vi "Folder Hierarchy Verifier.vi"() -> ()   [LabVIEW 2023]
doc: "Presents an interface to view the expected folder hierarchy on disk and and compare it to the actual folder hierarchy."
uses:
  CTLs/Folder Verifier State Data.ctl
  <userlib>/_MGI/Application Control/MGI Gray if/MGI Gray if False.vi
  SubVIs/FaKI State Machine/FaKI State Machine.lvlib
panel:
  in  "Project Hierarchy":string(tree)
  in  "Analyze Project":bool
  in  "Exit":bool
  in  "Project File":path
  # "A non-container project item will be red if expected path does not match actual path. A container project item will be red if none of the containing expected paths match actual paths, and purple if some match and some don't match"
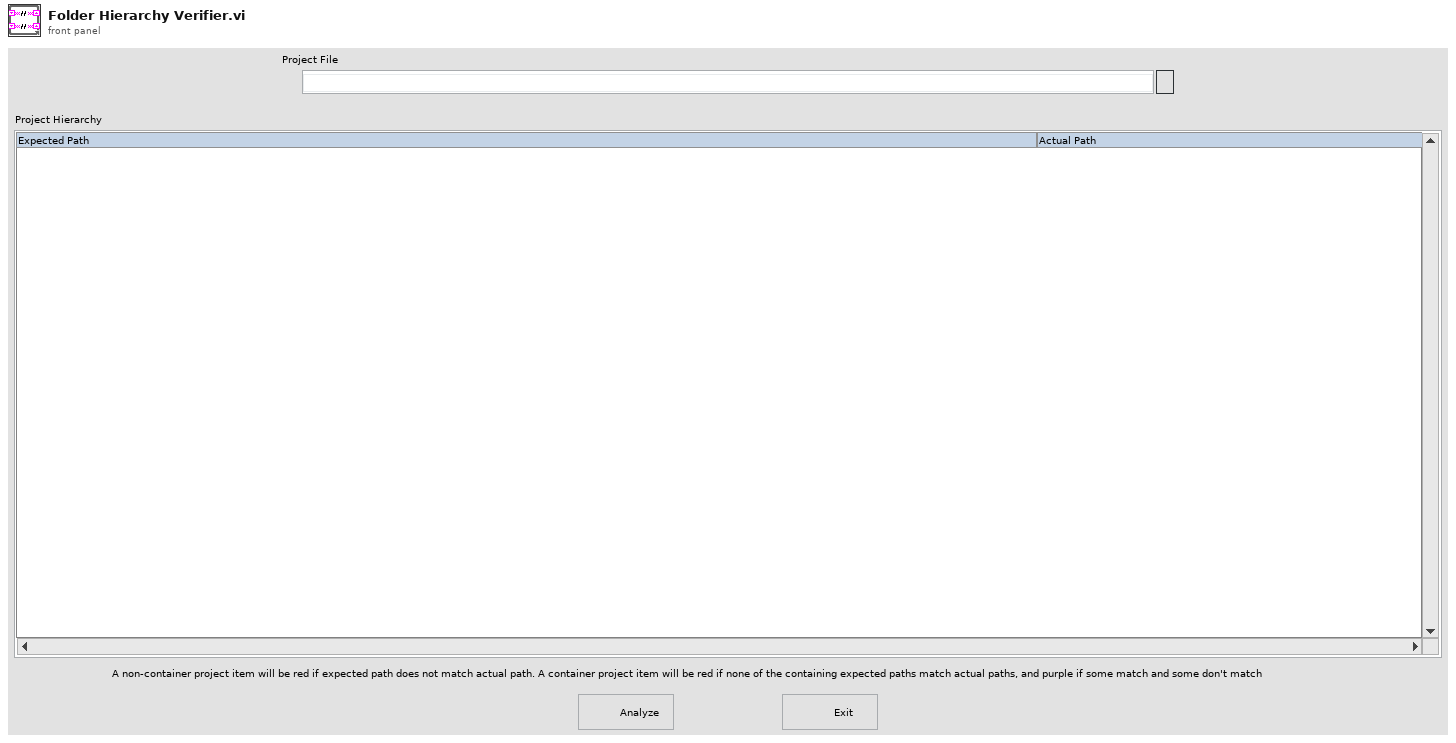
[diagram p1: front panel]
types:
  T1 = typedef "Folder Verifier State Data.ctl" = cluster{"Core":cluster{"Current VI Reference":refnum<vi>, "Close Panel on Exit?":bool}, "Tree Refnum":refnum<vi>, "Project":path, "Expected Paths":path[], "Actual Paths":path[]}
  T2 = enum32{"Invalid", "Standard", "Closed", "Hidden", "Minimized", "Maximized"}
  T3 = enum32{"invalid app kind", "Development System", "Run Time System", "Student Edition", "Embedded LabVIEW", "Evaluation", "Custom"}
  T4 = enum8{"Enabled", "Disabled", "Disabled and Grayed Out"}
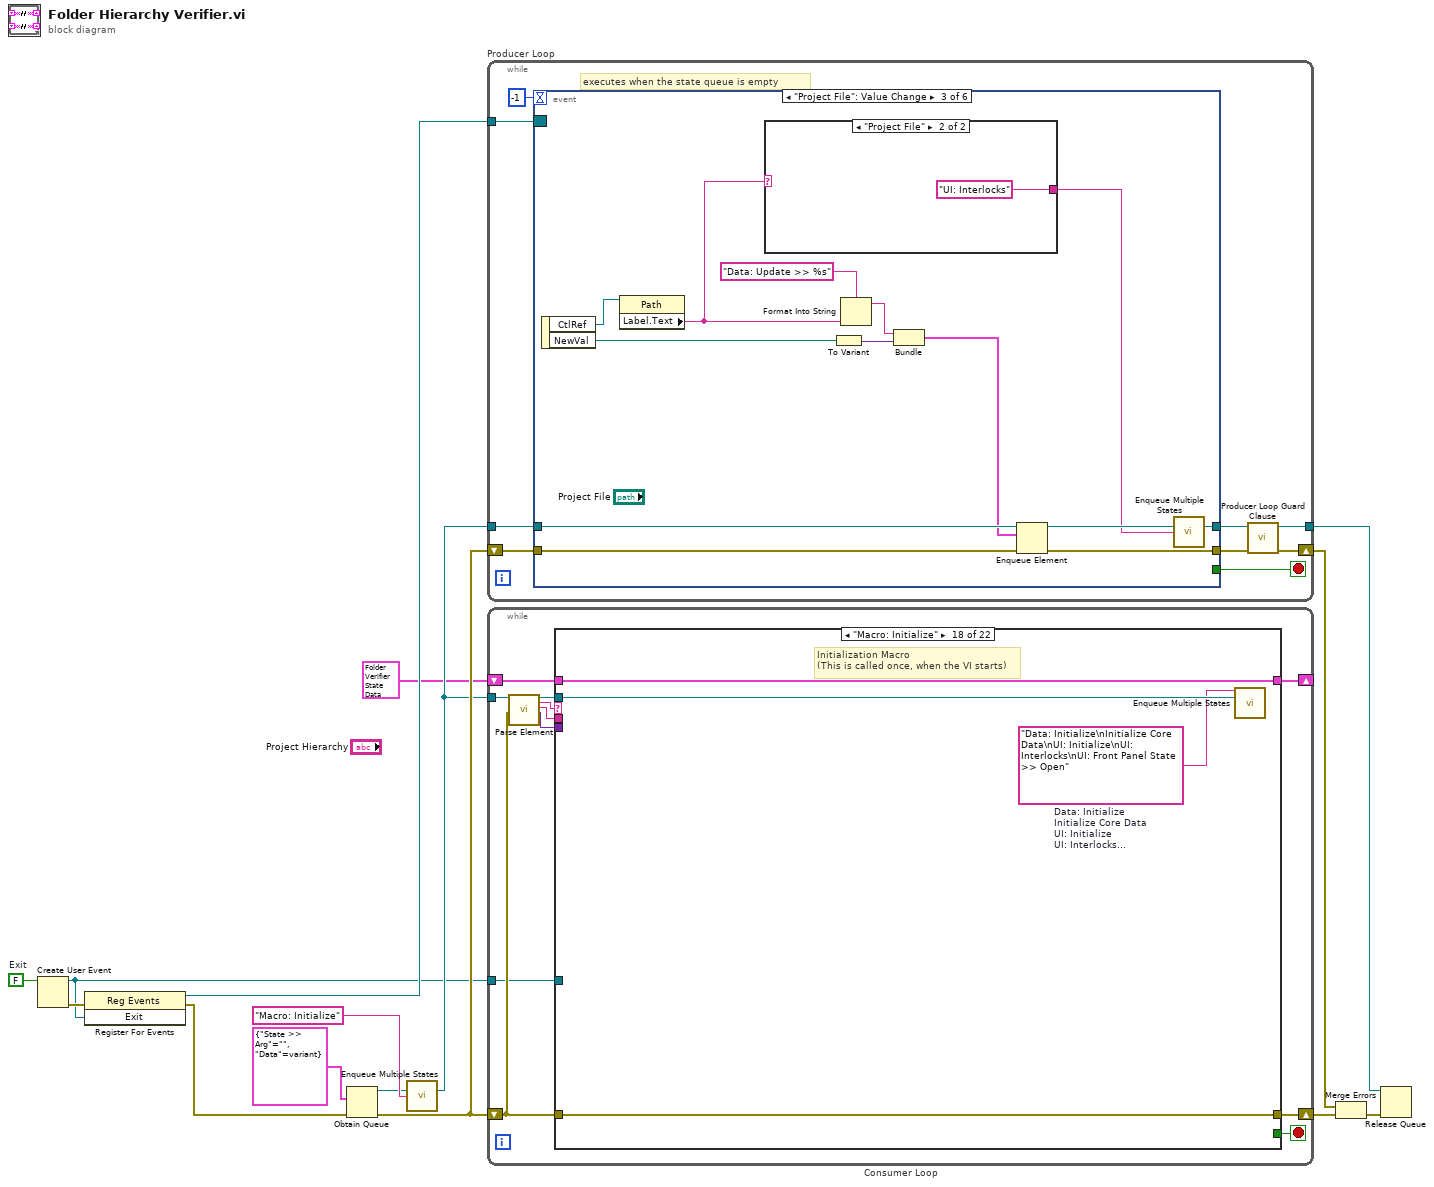
[diagram p0: block diagram]
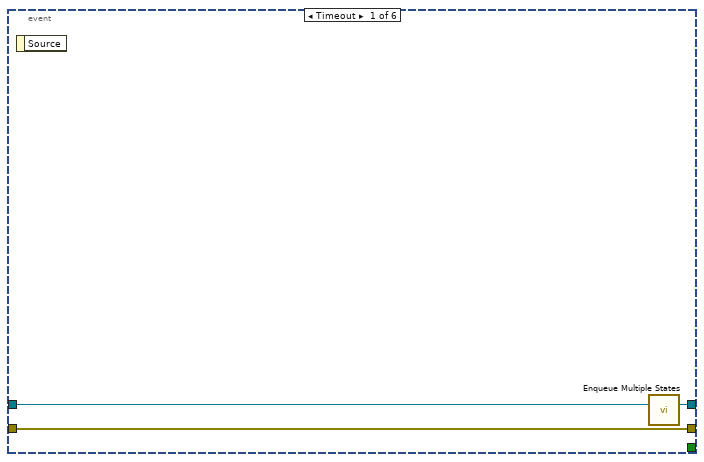
[diagram p2: hidden frame]
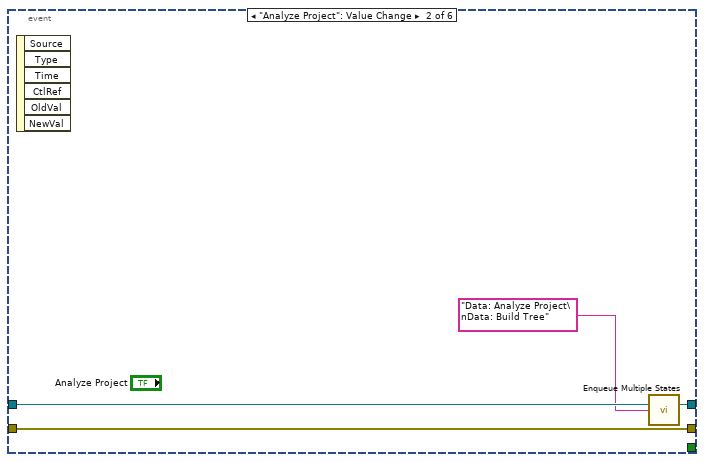
[diagram p3: hidden frame]
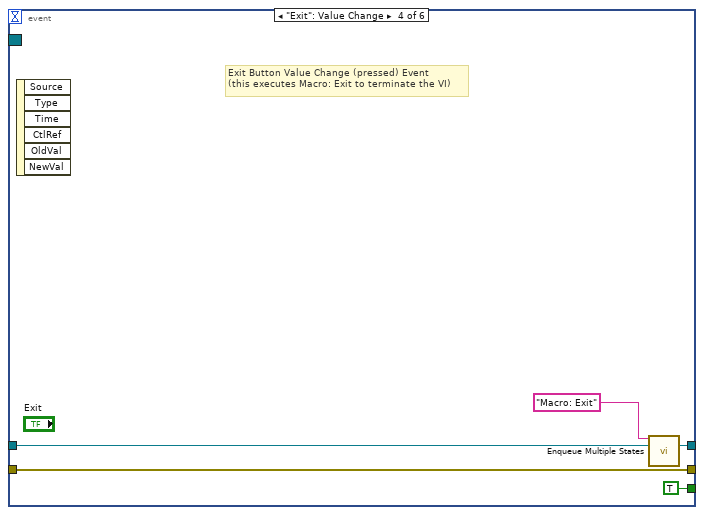
[diagram p5: hidden frame]
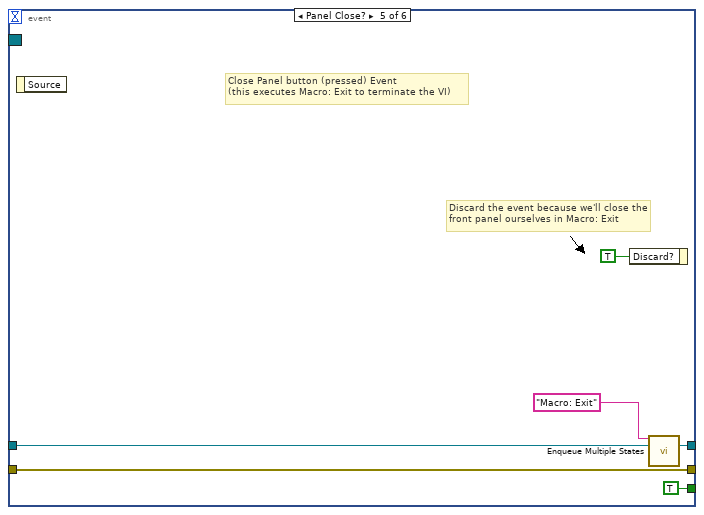
[diagram p6: hidden frame]
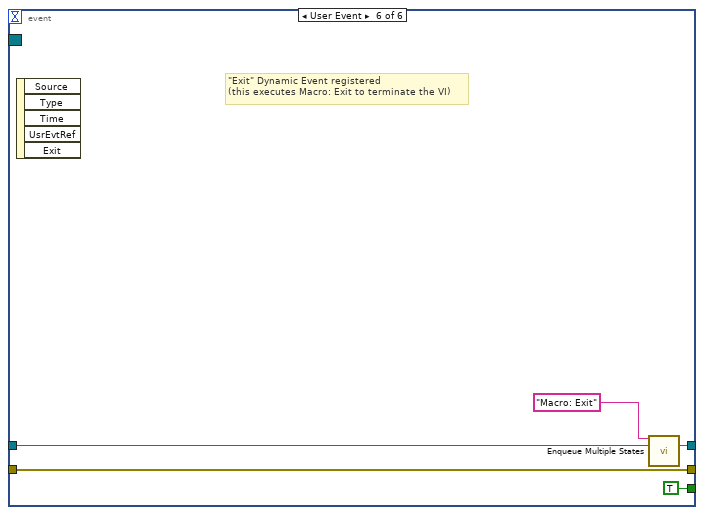
[diagram p7: hidden frame]
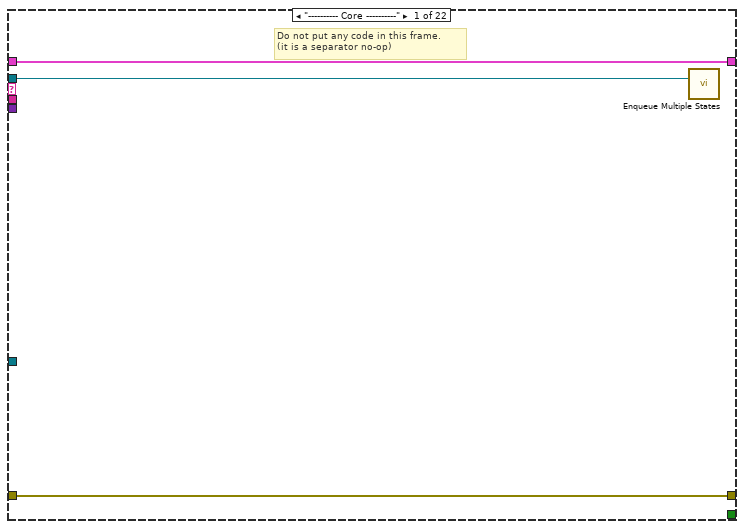
[diagram p8: hidden frame]
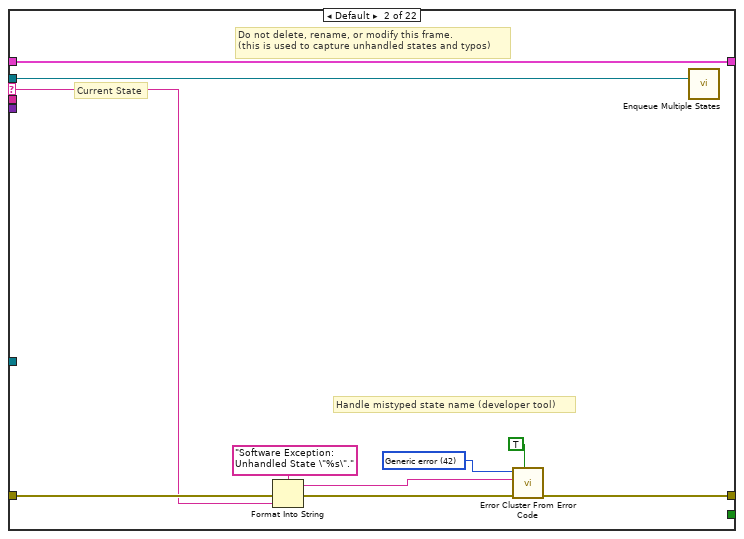
[diagram p9: hidden frame]
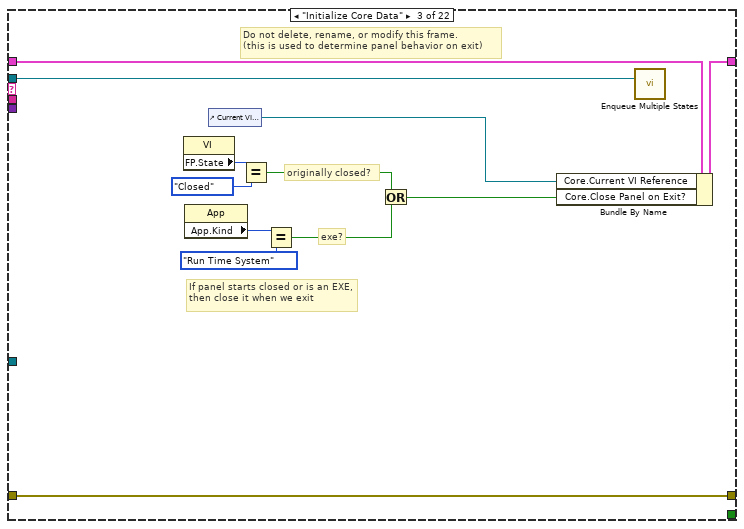
[diagram p10: hidden frame]
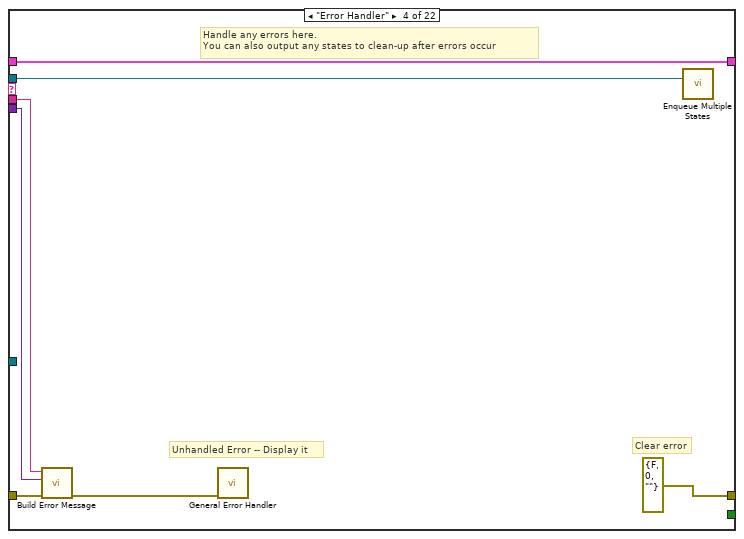
[diagram p11: hidden frame]
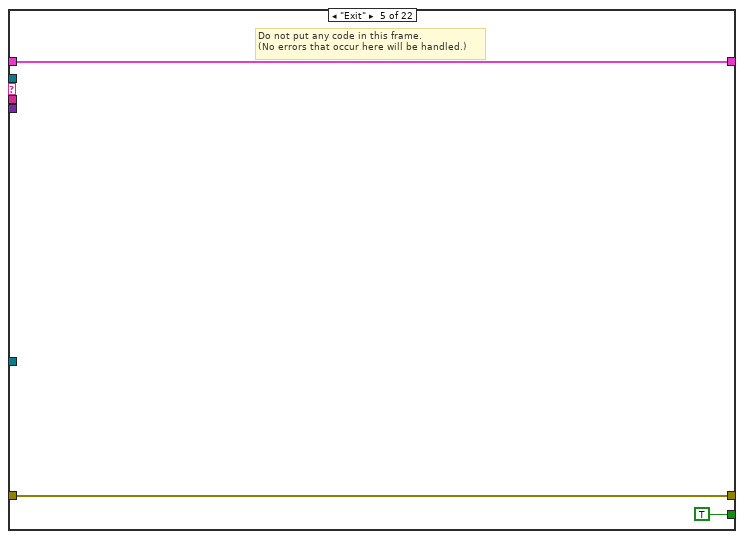
[diagram p12: hidden frame]
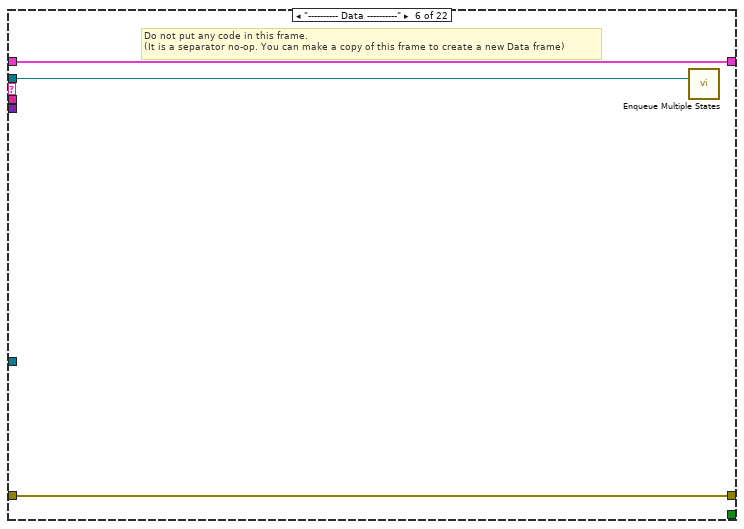
[diagram p13: hidden frame]
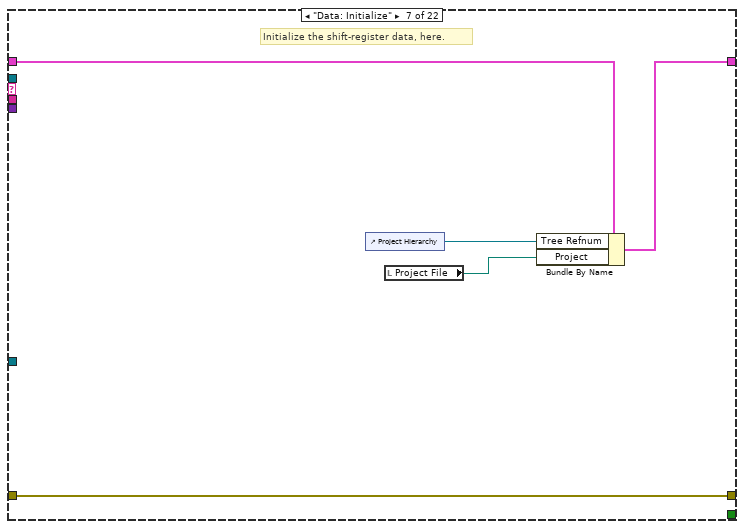
[diagram p14: hidden frame]
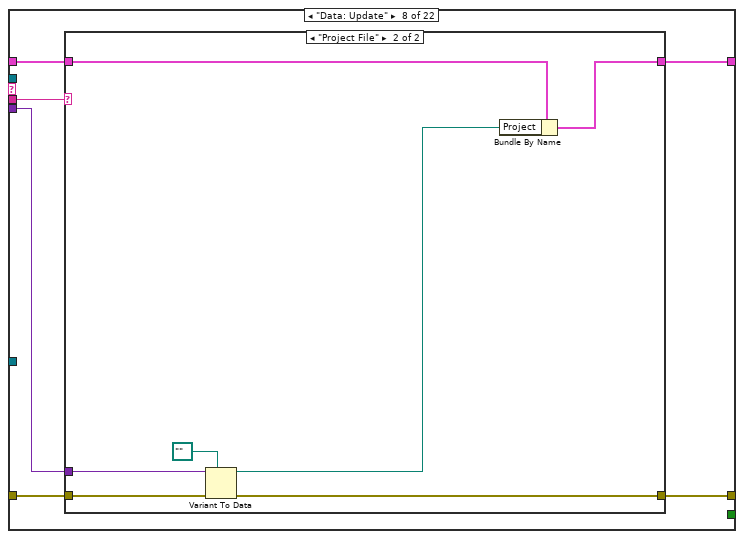
[diagram p15: hidden frame]
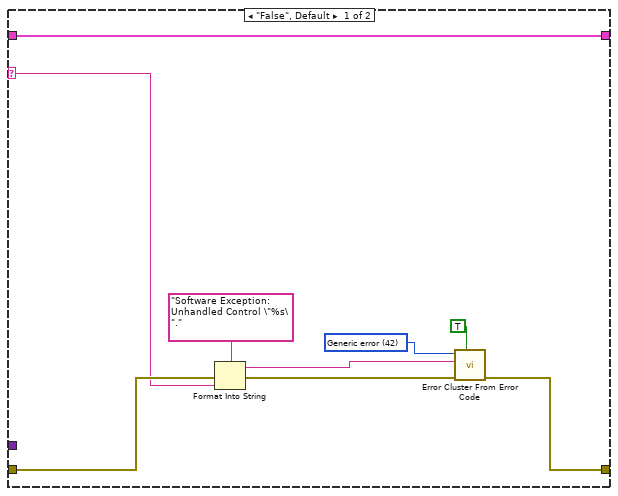
[diagram p16: hidden frame]
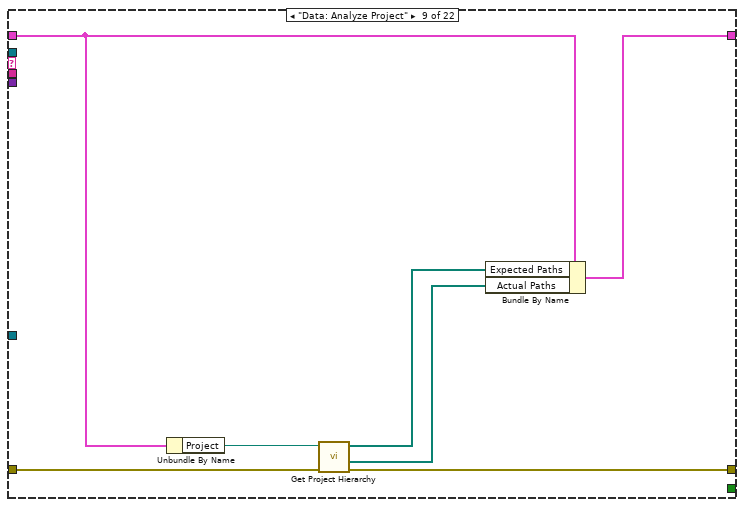
[diagram p17: hidden frame]
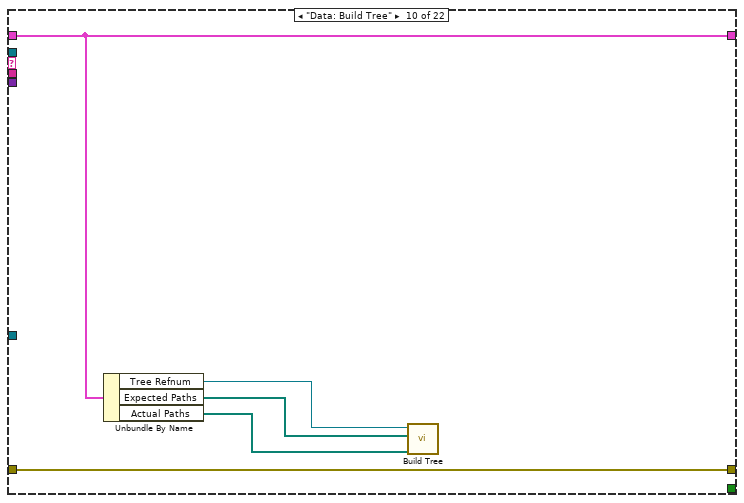
[diagram p18: hidden frame]
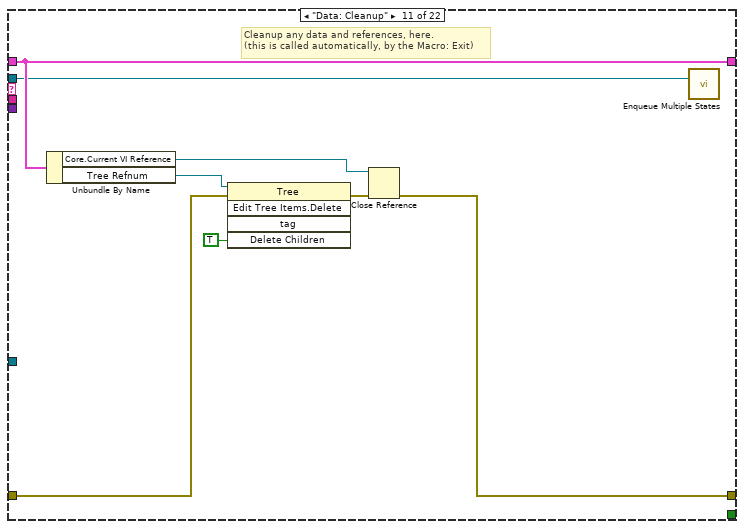
[diagram p19: hidden frame]
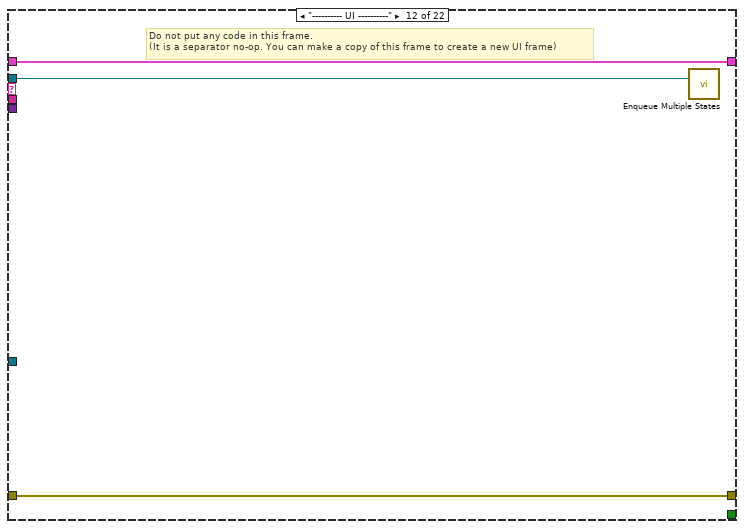
[diagram p20: hidden frame]
diagram:
  w5 = FALSE  # Exit
  n1 = Create User Event(user event datatype=w5) -> (user event=w2:refnum<user-event>, error out=w6:errorcluster)  [unwired: 1 in]
  n2 = register-events(error in=w6, w2) -> (reference out=w3:refnum<event-registration>, error out=w4:errorcluster)  [unwired: 1 in]
  n3 = Obtain Queue(element data type=cluster{"State >> Arg":string, "Data":variant} {"State >> Arg"="", "Data"=variant}, error in (no error)=w4) -> (queue out=w12:refnum<queue>, error out=w15:errorcluster)  [unwired: 3 in, 1 out]
  n4 = call "Enqueue Multiple States.vi"("queue in"=w12, "State(s) at Back"="Macro: Initialize") -> ("queue out"=w11:refnum<queue>)  [unwired: 13 in]
  n5 = while "Producer Loop" {
    shift-right: [w19] -> w9
    shift-left: w15 -> [w24]
    tunnel: w3 -> [w16]
    tunnel: w11 -> [w22]
    tunnel: [w17] -> w7
    stop <- w21 stop-if-true
    # "executes when the state queue is empty"
    n6 = event shown="[2] \"Project File\": Value Change" {
      selector: w16 -> [_ _ _ _ _ _]
      dyn-events: _ -> [_ _ _ _ _ _]
      timeout: -1 ("Timeout") -> [_ _ _ _ _ _]
      tunnel: [w25 w29 w42 w50 w56 w61] -> w20
      tunnel: w24 -> [w25 w29 w43 w50 w56 w61]
      tunnel: w22 -> [w26 w30 w41 w49 w53 w59]
      tunnel: [w27 w31 w44 w47 w52 w58] -> w18
      tunnel: [_ _ _ TRUE TRUE TRUE] -> w21
      event Timeout {
        n7 = event-data() -> ()  [unwired: 1 in, 1 out]
        n8 = call "Enqueue Multiple States.vi"("queue in"=w26) -> ("queue out"=w27:refnum<queue>)  [unwired: 14 in]
      }
      event "Analyze Project": Value Change {
        n9 = event-data() -> ()  [unwired: 1 in, 6 out]
        n10 = call "Enqueue Multiple States.vi"("queue in"=w30, "State(s) at Back"="Data: Analyze Project\nData: Build Tree") -> ("queue out"=w31:refnum<queue>)  [unwired: 13 in]
      }
      event "Project File": Value Change {
        n11 = event-data() -> ("CtlRef"=w39:refnum<vi>, "NewVal"=w38:path)  [unwired: 1 in]
        n12 = property class="Path"(reference=w39) -> ("Label.Text"=w34:string)  [unwired: 1 in, 2 out]
        n13 = case shown="\"Project File\"" w34 {
          tunnel: [_ "UI: Interlocks"] -> w32
          frame "False", Default {
          }
          frame "Project File" {
          }
        }
        n14 = To Variant(anything=w38) -> (Variant=w37:variant)
        n15 = Format Into String(format string="Data: Update >> %s", w34) -> (resulting string=w36:string)  [unwired: 2 in, 1 out]
        n16 = Bundle(w36, "Variant"=w37) -> (w33:cluster{string, "Variant":variant})  [unwired: 1 in]
        n17 = Enqueue Element(queue=w41, element=w33, error in (no error)=w43) -> (queue out=w40:refnum<queue>, error out=w42:errorcluster)  [unwired: 1 in, 1 out]
        n18 = call "Enqueue Multiple States.vi"("queue in"=w40, "State(s) at Back"=w32) -> ("queue out"=w44:refnum<queue>)  [unwired: 13 in]
      }
      event "Exit": Value Change {
        # "Exit Button Value Change (pressed) Event\n(this executes Macro: Exit to terminate the VI)"
        n19 = event-data() -> ()  [unwired: 1 in, 6 out]
        n20 = call "Enqueue Multiple States.vi"("State(s) at Front"="Macro: Exit", "queue in"=w49) -> ("queue out"=w47:refnum<queue>)  [unwired: 13 in]
      }
      event Panel Close? {
        # "Discard the event because we'll close the front panel ourselves in Macro: Exit"
        # "Close Panel button (pressed) Event\n(this executes Macro: Exit to terminate the VI)"
        n21 = event-data() -> ()  [unwired: 1 in, 1 out]
        n22 = event-data("Discard?"=TRUE) -> ()  [unwired: 1 in, 1 out]
        n23 = call "Enqueue Multiple States.vi"("State(s) at Front"="Macro: Exit", "queue in"=w53) -> ("queue out"=w52:refnum<queue>)  [unwired: 13 in]
      }
      event User Event {
        # "\"Exit\" Dynamic Event registered\n(this executes Macro: Exit to terminate the VI)"
        n24 = event-data() -> ()  [unwired: 1 in, 5 out]
        n25 = call "Enqueue Multiple States.vi"("State(s) at Front"="Macro: Exit", "queue in"=w59) -> ("queue out"=w58:refnum<queue>)  [unwired: 13 in]
      }
    }
    n26 = call "Producer Loop Guard Clause.vi"("error in (no error)"=w20, "queue in"=w18) -> ("error out"=w19:errorcluster, "queue out"=w17:refnum<queue>)  [unwired: 8 in]
  }
  n27 = while "Consumer Loop" {
    shift-right: [w69] -> _
    shift-left: T1 {"Core"={"Current VI Reference"=refnum, "Close Panel on Exit?"=FALSE}, "Tree Refnum"=refnum, "Project"=path "", "Expected Paths"=[], "Actual Paths"=[]} ("Folder Verifier State Data") -> [w68]
    shift-right: [w72] -> w10
    shift-left: w15 -> [w71]
    tunnel: w11 -> [w67]
    tunnel: w2 -> [w62]
    stop <- w70 stop-if-true
    n28 = call "Parse Element.vi"("queue in"=w67, "error in (no error)"=w71) -> ("queue out"=w66:refnum<queue>, "State"=w65:string, "Arg"=w64:string, "Data"=w63:variant)  [unwired: 14 in]
    n29 = case shown="\"Macro: Initialize\"" w65 {
      selector: w65 -> [_ w77 _ _ _ _ _ _ _ _ _ _ _ _ _ _ _ _ _ _ _ _]
      tunnel: w66 -> [w73 w76 w86 w102 _ w108 _ _ _ _ w154 w158 w161 _ w170 w179 w250 w254 w260 w266 w269 w272]
      tunnel: w64 -> [_ _ _ w98 _ _ _ w119 _ _ _ _ _ _ w171 w180 _ _ _ _ _ _]
      tunnel: w68 -> [w74 w79 w92 w103 w106 w109 w114 w120 w139 w149 w155 w159 w162 w168 w172 w182 w251 w255 w264 w267 w270 w273]
      tunnel: [w75 w84 w97 errorcluster {"status"=FALSE, "code"=0, "source"=""} ("error out") w107 w110 w115 w117 w143 w148 w157 w160 w163 w169 w173 w183 w252 w256 w265 w268 w271 w274] -> w72
      tunnel: w71 -> [w75 w83 w97 w101 w107 w110 w115 w121 w144 w148 w151 w160 w163 w169 w174 w184 w252 w256 w265 w268 w271 w274]
      tunnel: [_ _ _ _ TRUE _ _ _ _ _ _ _ _ _ _ _ _ _ _ _ _ _] -> w70
      tunnel: [w74 w79 w96 w103 w106 w109 w113 w116 w142 w149 w155 w159 w162 w168 w172 w182 w251 w255 w264 w267 w270 w273] -> w69
      tunnel: w63 -> [_ _ _ w99 _ _ _ w118 _ _ _ _ _ _ _ _ _ _ _ _ _ _]
      tunnel: w62 -> [_ _ _ _ _ _ _ _ _ _ _ _ _ _ _ _ _ _ _ _ _ _]
      frame "---------- Core ----------" {
        # "Do not put any code in this frame.\n(it is a separator no-op)"
        n30 = call "Enqueue Multiple States.vi"("queue in"=w73) -> ()  [unwired: 14 in, 1 out]
      }
      frame Default {
        w81 = 42 items=["No error", "Argument error", "Memory is full", "Out of zone", "End of file", "File already open", "Generic file I/O error", "File not found", "File permission error", "Disk is full", "Duplicate path", "Too many files open", "System feature not enabled", "Resource file not found", "Cannot add resource", "Resource not found", "Image not found", "Image memory error", "Pen does not exist", "Config type invalid", "Config token not found", "Config parse error", "Config memory error", "Bad external code format", "Bad external code offset", "External code not present", "Null window", "Destroy window error", "Null menu", "Print aborted", "Bad print record", "Print driver error", "Windows error during printing", "Memory error during printing", "Print dialog error", "Generic print error", "Invalid device refnum", "Device not found", "Device parameter error", "Device unit error", "Cannot open device", "Device call aborted", "Generic error", "Cancelled by user", "Object ID too low", "Object ID too high", "Object not in heap", "Unknown heap", "Unknown object (invalid DefProc)", "Unknown object (DefProc not in table)", "Message out of range", "Invalid (null) method", "Unknown message", "Manager call not supported", "Bad address", "Network operation in progress", "Network operation timed out", "Connection is busy", "Network attribute not supported", "Network error", "Address in use", "System out of memory", "Connection aborted", "Connection refused", "Not connected", "Already connected", "Connection closed", "Initialization error (interapplication manager)", "Bad occurrence", "Wait on unbound occurrence handler", "Occurrence queue overflow", "Datalog type conflict", "Unused", "Unrecognized type (interapplication manager)", "Memory corrupt", "Failed to make temporary DLL", "Old CIN version", "Drag socket not found", "Failed to load drop-object", "Failed to register OLE object", "Failed to release OLE object", "Format specifier type mismatch", "Unknown format specifier", "Too few format specifiers", "Too many format specifiers", "Scan failed", "Newer CIN version", "Error converting to variant", "Runtime menu error", "Password tampered", "Variant attribute not found", "Incompatible variant data type", "Event data is not available", "Event Store is not present", "Occurrence is not found", "Event Queue is not created", "Event info is not available", "Refnum passed is NULL", "Error retrieving Class GUID", "Error retrieving CoClass GUID", "Error retrieving TypeLib GUID.", "Bad built application magic bytes.", "Specific driver is different from the specific driver associated with the Logical Name.", "There is no session opened to the class driver.", "Max Error", "MAX - Error with config objects", "MAX - Error loading configuration", "MAX - Group not supported"]
        # "Current State"
        # "Do not delete, rename, or modify this frame.\n(this is used to capture unhandled states and typos)"
        # "Handle mistyped state name (developer tool)"
        n31 = Format Into String(format string="Software Exception: Unhandled State \"%s\"." ("message"), error in=w83, w77) -> (resulting string=w80:string, error out=w85:errorcluster)  [unwired: 1 in]
        n32 = call <vilib>:"Error Cluster From Error Code.vi"("show call chain? (False)"=TRUE, "error in (no error)"=w85, "error message (\"\")"=w80, "error code (0)"=w81) -> ("error out"=w84:errorcluster)  [unwired: 5 in]
        n33 = call "Enqueue Multiple States.vi"("queue in"=w76) -> ()  [unwired: 14 in, 1 out]
      }
      frame "Initialize Core Data" {
        # "Do not delete, rename, or modify this frame.\n(this is used to determine panel behavior on exit)"
        # "originally closed?"
        # "exe?"
        # "If panel starts closed or is an EXE, then close it when we exit"
        n34 = property class="VI"() -> ("FP.State"=w89:T2)  [unwired: 2 in, 2 out]
        n35 = property class="App"() -> ("App.Kind"=w95:T3)  [unwired: 2 in, 2 out]
        n36 = control-ref of="Current VI Reference"() -> (w90:refnum<vi>)
        n37 = Equal?(x=w89, y=T2."Closed" ("Front Panel Window:State")) -> (x = y?=w87:bool)
        n38 = Equal?(x=w95, y=T3."Run Time System" ("Application:Kind")) -> (x = y?=w93:bool)
        n39 = Or(x=w87, y=w93) -> (x .or. y?=w91:bool)
        n40 = Bundle By Name(cluster=w92, "Core.Current VI Reference"=w90, "Core.Close Panel on Exit?"=w91) -> (w96:T1)
        n41 = call "Enqueue Multiple States.vi"("queue in"=w86) -> ()  [unwired: 14 in, 1 out]
      }
      frame "Error Handler" {
        # "Unhandled Error -- Display it"
        # "Handle any errors here.\nYou can also output any states to clean-up after errors occur"
        # "Clear error"
        n42 = call "Build Error Message.vi"("error in (no error)"=w101, "Data"=w99, "Arg"=w98) -> ("error out"=w100:errorcluster)  [unwired: 8 in]
        n43 = call <vilib>:"General Error Handler.vi"("error in (no error)"=w100) -> ()  [unwired: 10 in, 5 out]
        n44 = call "Enqueue Multiple States.vi"("queue in"=w102) -> ()  [unwired: 14 in, 1 out]
      }
      frame "Exit" {
        # "Do not put any code in this frame.\n(No errors that occur here will be handled.)"
      }
      frame "---------- Data ----------" {
        # "Do not put any code in this frame.\n(It is a separator no-op. You can make a copy of this frame to create a new Data frame)"
        n45 = call "Enqueue Multiple States.vi"("queue in"=w108) -> ()  [unwired: 14 in, 1 out]
      }
      frame "Data: Initialize" {
        # "Initialize the shift-register data, here."
        n46 = control-ref of="Project Hierarchy"() -> (w112:refnum<vi>)
        n47 = local read "Project File"() -> (w111:path)
        n48 = Bundle By Name(cluster=w114, "Tree Refnum"=w112, "Project"=w111) -> (w113:T1)
      }
      frame "Data: Update" {
        n49 = case shown="\"Project File\"" w119 {
          selector: w119 -> [w122 _]
          tunnel: w121 -> [w124 w136]
          tunnel: w120 -> [w130 w133]
          tunnel: w118 -> [_ w137]
          tunnel: [w123 w134] -> w117
          tunnel: [w130 w132] -> w116
          frame "False", Default {
            w128 = 42 items=["No error", "Argument error", "Memory is full", "Out of zone", "End of file", "File already open", "Generic file I/O error", "File not found", "File permission error", "Disk is full", "Duplicate path", "Too many files open", "System feature not enabled", "Resource file not found", "Cannot add resource", "Resource not found", "Image not found", "Image memory error", "Pen does not exist", "Config type invalid", "Config token not found", "Config parse error", "Config memory error", "Bad external code format", "Bad external code offset", "External code not present", "Null window", "Destroy window error", "Null menu", "Print aborted", "Bad print record", "Print driver error", "Windows error during printing", "Memory error during printing", "Print dialog error", "Generic print error", "Invalid device refnum", "Device not found", "Device parameter error", "Device unit error", "Cannot open device", "Device call aborted", "Generic error", "Cancelled by user", "Object ID too low", "Object ID too high", "Object not in heap", "Unknown heap", "Unknown object (invalid DefProc)", "Unknown object (DefProc not in table)", "Message out of range", "Invalid (null) method", "Unknown message", "Manager call not supported", "Bad address", "Network operation in progress", "Network operation timed out", "Connection is busy", "Network attribute not supported", "Network error", "Address in use", "System out of memory", "Connection aborted", "Connection refused", "Not connected", "Already connected", "Connection closed", "Initialization error (interapplication manager)", "Bad occurrence", "Wait on unbound occurrence handler", "Occurrence queue overflow", "Datalog type conflict", "Unused", "Unrecognized type (interapplication manager)", "Memory corrupt", "Failed to make temporary DLL", "Old CIN version", "Drag socket not found", "Failed to load drop-object", "Failed to register OLE object", "Failed to release OLE object", "Format specifier type mismatch", "Unknown format specifier", "Too few format specifiers", "Too many format specifiers", "Scan failed", "Newer CIN version", "Error converting to variant", "Runtime menu error", "Password tampered", "Variant attribute not found", "Incompatible variant data type", "Event data is not available", "Event Store is not present", "Occurrence is not found", "Event Queue is not created", "Event info is not available", "Refnum passed is NULL", "Error retrieving Class GUID", "Error retrieving CoClass GUID", "Error retrieving TypeLib GUID.", "Bad built application magic bytes.", "Specific driver is different from the specific driver associated with the Logical Name.", "There is no session opened to the class driver.", "Max Error", "MAX - Error with config objects", "MAX - Error loading configuration", "MAX - Group not supported"]
            n50 = Format Into String(format string="Software Exception: Unhandled Control \"%s\"." ("message"), error in=w124, w122) -> (resulting string=w127:string, error out=w129:errorcluster)  [unwired: 1 in]
            n51 = call <vilib>:"Error Cluster From Error Code.vi"("show call chain? (False)"=TRUE, "error in (no error)"=w129, "error message (\"\")"=w127, "error code (0)"=w128) -> ("error out"=w123:errorcluster)  [unwired: 5 in]
          }
          frame "Project File" {
            n52 = Variant To Data(error in=w136, type=path "", Variant=w137) -> (data=w131:path, error out=w134:errorcluster)
            n53 = Bundle By Name(cluster=w133, "Project"=w131) -> (w132:T1)
          }
        }
      }
      frame "Data: Analyze Project" {
        n54 = Unbundle By Name(w139) -> ("Project"=w138:path)
        n55 = call "Get Project Hierarchy.vi"("error in (no error)"=w144, "Project Path"=w138) -> ("error out"=w143:errorcluster, "Actual Locations"=w140:path[], "Expected Locations"=w141:path[])  [unwired: 7 in]
        n56 = Bundle By Name(cluster=w139, "Expected Paths"=w141, "Actual Paths"=w140) -> (w142:T1)
      }
      frame "Data: Build Tree" {
        n57 = Unbundle By Name(w149) -> ("Tree Refnum"=w145:refnum<vi>, "Expected Paths"=w146:path[], "Actual Paths"=w147:path[])
        n58 = call "Build Tree.vi"("Actual Path"=w147, "Expected Path"=w146, "Tree Refnum"=w145) -> ()  [unwired: 9 in]
      }
      frame "Data: Cleanup" {
        # "Cleanup any data and references, here.\n(this is called automatically, by the Macro: Exit)"
        n59 = Unbundle By Name(w155) -> ("Core.Current VI Reference"=w156:refnum<vi>, "Tree Refnum"=w153:refnum<vi>)
        n60 = invoke class="Tree" method="Edit Tree Items.Delete"(reference=w153, error in=w151, "Delete Children"=TRUE ("Delete Children?")) -> (error out=w150:errorcluster)  [unwired: 2 in, 4 out]
        n61 = Close Reference(reference=w156, error in (no error)=w150) -> (error out=w157:errorcluster)
        n62 = call "Enqueue Multiple States.vi"("queue in"=w154) -> ()  [unwired: 14 in, 1 out]
      }
      frame "---------- UI ----------" {
        # "Do not put any code in this frame.\n(It is a separator no-op. You can make a copy of this frame to create a new UI frame)"
        n63 = call "Enqueue Multiple States.vi"("queue in"=w158) -> ()  [unwired: 14 in, 1 out]
      }
      frame "UI: Initialize" {
        # "Initialize the User Interface, here.\n(this is called automatically, by the Macro: Init)"
        n64 = call "Enqueue Multiple States.vi"("queue in"=w161) -> ()  [unwired: 14 in, 1 out]
      }
      frame "UI: Interlocks" {
        n65 = Unbundle By Name(w168) -> ("Project"=w165:path)
        n66 = Empty String/Path?(string/path=w165) -> (empty?=w166:bool)
        n67 = Not(x=w166) -> (.not. x?=w164:bool)
        n68 = call-poly <userlib>:"MGI Gray if.vi"("Boolean"=w164) -> ("Disabled"=w167:T4)
        n69 = property on="Analyze Project" class="Bool"("DisabledEnum"=w167) -> ()  [unwired: 2 in, 2 out]
      }
      frame "UI: Cursor Set" {
        # "Argument"
        # "Set and Unset Cursor Busy.\n(Usage: \"UI: Cursor Set >> Busy|Idle\")"
        n70 = case shown="\"Idle\", Default" w171 {
          tunnel: w174 -> [w176 w178]
          tunnel: [w175 w177] -> w173
          frame "Idle", Default {
            n71 = call <vilib>:"Unset Busy.vi"("error in (no error)"=w176) -> ("error out"=w175:errorcluster)  [unwired: 10 in]
          }
          frame "Busy" {
            n72 = call <vilib>:"Set Busy.vi"("error in (no error)"=w178) -> ("error out"=w177:errorcluster)  [unwired: 9 in, 1 out]
          }
        }
        n73 = call "Enqueue Multiple States.vi"("queue in"=w170) -> ()  [unwired: 14 in, 1 out]
      }
      frame "UI: Front Panel State" {
        # "Argument"
        # "Set Front Panel Open or Closed\n(Usage: \"UI: Front Panel State >> Open|Close\")"
        n74 = Unbundle By Name(w182) -> ("Core.Current VI Reference"=w181:refnum<vi>)
        n75 = case shown="\"Open\", \"Standard\", Default" w180 {
          tunnel: w184 -> [w191 w205 w217 w230 w243]
          tunnel: [w192 w206 w218 w231 w244] -> w183
          tunnel: w181 -> [w189 w203 w215 w228 w241]
          frame "Open", "Standard", Default {
            w185 = T2."Standard" ("State")
            n76 = property class="VI"(reference=w189, error in=w191) -> (reference out=w188:refnum<vi>, error out=w190:errorcluster, "FP.State"=w187:T2)
            n77 = Not Equal?(x=w187, y=w185) -> (x != y?=w186:bool)
            n78 = case shown="True" w186 {
              tunnel: [w197 w198] -> w192
              tunnel: w190 -> [w196 w198]
              tunnel: w188 -> [w194 _]
              tunnel: w185 -> [w193 _]
              frame True {
                n79 = invoke class="VI" method="FP.Open"(reference=w194, error in=w196, "Activate"=TRUE, "State"=w193) -> (error out=w197:errorcluster)  [unwired: 1 in, 4 out]
              }
              frame False {
              }
            }
          }
          frame "Close", "Closed" {
            n80 = property class="VI"(reference=w203, error in=w205) -> (reference out=w202:refnum<vi>, error out=w204:errorcluster, "FP.State"=w200:T2)
            n81 = Not Equal?(x=w200, y=T2."Closed" ("Front Panel Window:State")) -> (x != y?=w199:bool)
            n82 = case shown="True" w199 {
              tunnel: [w207 w210] -> w206
              tunnel: w204 -> [w207 w209]
              tunnel: w202 -> [_ w208]
              frame False {
              }
              frame True {
                n83 = invoke class="VI" method="FP.Close"(reference=w208, error in=w209) -> (error out=w210:errorcluster)  [unwired: 1 in, 2 out]
              }
            }
          }
          frame "Hidden", "Hide" {
            w211 = T2."Hidden" ("State")
            n84 = property class="VI"(reference=w215, error in=w217) -> (reference out=w214:refnum<vi>, error out=w216:errorcluster, "FP.State"=w213:T2)
            n85 = Not Equal?(x=w213, y=w211) -> (x != y?=w212:bool)
            n86 = case shown="True" w212 {
              tunnel: [w222 w223] -> w218
              tunnel: w216 -> [w221 w223]
              tunnel: w214 -> [w220 _]
              tunnel: w211 -> [w219 _]
              frame True {
                n87 = invoke class="VI" method="FP.Open"(reference=w220, error in=w221, "State"=w219) -> (error out=w222:errorcluster)  [unwired: 2 in, 4 out]
              }
              frame False {
              }
            }
          }
          frame "Minimize", "Minimized" {
            w224 = T2."Minimized" ("State")
            n88 = property class="VI"(reference=w228, error in=w230) -> (reference out=w227:refnum<vi>, error out=w229:errorcluster, "FP.State"=w226:T2)
            n89 = Not Equal?(x=w226, y=w224) -> (x != y?=w225:bool)
            n90 = case shown="True" w225 {
              tunnel: [w235 w236] -> w231
              tunnel: w229 -> [w234 w236]
              tunnel: w227 -> [w233 _]
              tunnel: w224 -> [w232 _]
              frame True {
                n91 = invoke class="VI" method="FP.Open"(reference=w233, error in=w234, "State"=w232) -> (error out=w235:errorcluster)  [unwired: 2 in, 4 out]
              }
              frame False {
              }
            }
          }
          frame "Maximize", "Maximized" {
            w237 = T2."Maximized" ("State")
            n92 = property class="VI"(reference=w241, error in=w243) -> (reference out=w240:refnum<vi>, error out=w242:errorcluster, "FP.State"=w239:T2)
            n93 = Not Equal?(x=w239, y=w237) -> (x != y?=w238:bool)
            n94 = case shown="True" w238 {
              tunnel: [w248 w249] -> w244
              tunnel: w242 -> [w247 w249]
              tunnel: w240 -> [w246 _]
              tunnel: w237 -> [w245 _]
              frame True {
                n95 = invoke class="VI" method="FP.Open"(reference=w246, error in=w247, "State"=w245) -> (error out=w248:errorcluster)  [unwired: 2 in, 4 out]
              }
              frame False {
              }
            }
          }
        }
        n96 = call "Enqueue Multiple States.vi"("queue in"=w179) -> ()  [unwired: 14 in, 1 out]
      }
      frame "---------- Macro ----------" {
        # "Do not put any code in this frame.\n(It is a separator no-op. You can make a copy of this frame to create a new Macro frame)"
        n97 = call "Enqueue Multiple States.vi"("queue in"=w250) -> ()  [unwired: 14 in, 1 out]
      }
      frame "Macro: Initialize" {
        w253 = "Data: Initialize\nInitialize Core Data\nUI: Initialize\nUI: Interlocks\nUI: Front Panel State >> Open"  # Data: Initialize Initialize Core Data UI: Initialize UI: Interlocks UI: Front Panel State >> Open
        # "Initialization Macro\n(This is called once, when the VI starts)"
        n98 = call "Enqueue Multiple States.vi"("State(s) at Front"=w253, "queue in"=w254) -> ()  [unwired: 13 in, 1 out]
      }
      frame "Macro: Exit" {
        # "Exit Macro\n(This is called once, when the VI exits)"
        n99 = Unbundle By Name(w264) -> ("Core.Close Panel on Exit?"=w263:bool)
        n100 = Select(t="UI: Front Panel State >> Close\n", s=w263, f="") -> (s? t:f=w259:string)
        n101 = Concatenate Strings(w259, "Data: Cleanup\nExit") -> (w257:string)
        n102 = call "Enqueue Multiple States.vi"("State(s) at Front"=w257, "queue in"=w260) -> ()  [unwired: 13 in, 1 out]
      }
      frame "---------- New Category ----------" {
        # "Template Separator\n(You can make a copy of, or modify, this frame)"
        n103 = call "Enqueue Multiple States.vi"("queue in"=w266) -> ()  [unwired: 14 in, 1 out]
      }
      frame "New Category: 1" {
        # "Your code here.\n(You can make a copy of, or modify, this frame)"
        n104 = call "Enqueue Multiple States.vi"("queue in"=w269) -> ()  [unwired: 14 in, 1 out]
      }
      frame "New Category: 2" {
        # "Your code here.\n(You can make a copy of, or modify, this frame)"
        n105 = call "Enqueue Multiple States.vi"("queue in"=w272) -> ()  [unwired: 14 in, 1 out]
      }
    }
  }
  n106 = Merge Errors(w9, w10) -> (w8:errorcluster)
  n107 = Release Queue(queue=w7, error in (no error)=w8) -> ()  [unwired: 1 in, 3 out]
